vi "Write Graph-Chart Plot Names.vi"(8 "error in":errorcluster, 10 "Value":string[](array[string]), 11 "Graph / Chart Reference in":refnum<vi>) -> (0 "error out":errorcluster, 3 "Graph / Chart Reference out":refnum<vi>)   [LabVIEW 2020, in "G-Unicode.lvlib"]
uses:
  G-Unicode.lvlib
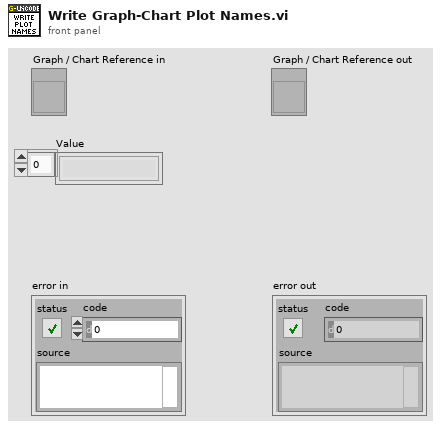
[diagram p1: front panel]
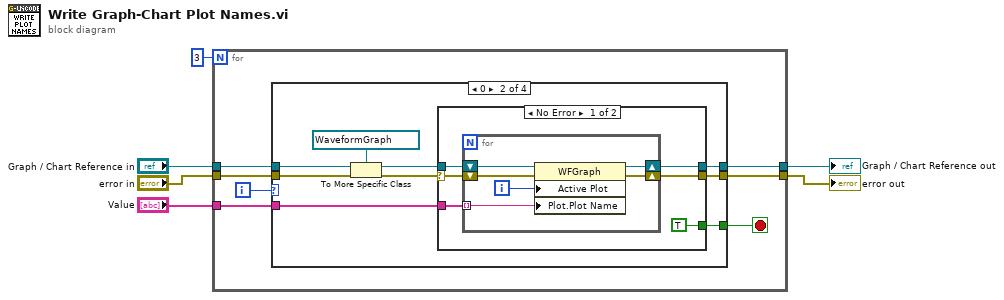
[diagram p0: block diagram]
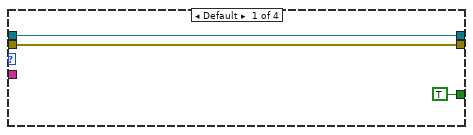
[diagram p2: hidden frame]
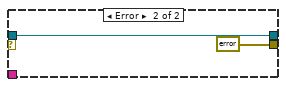
[diagram p3: hidden frame]
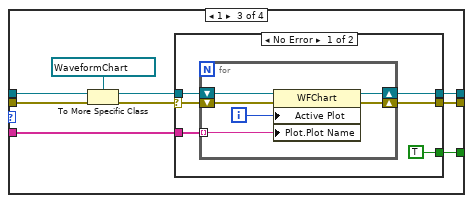
[diagram p4: hidden frame]
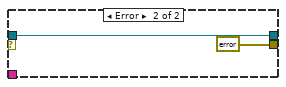
[diagram p5: hidden frame]
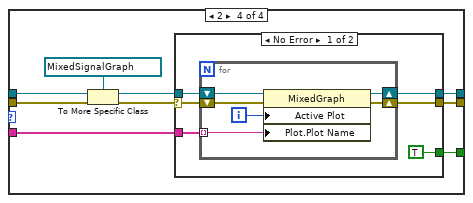
[diagram p6: hidden frame]
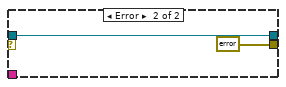
[diagram p7: hidden frame]
diagram:
  n1 = for {
    N: 3 -> [_]
    tunnel: "error in" -> [w13]
    tunnel: [w12] -> w5
    tunnel: [w11] -> w4
    tunnel: "Graph / Chart Reference in" -> [w10]
    tunnel: "Value" -> [w9]
    i -> [w8]
    stop <- w7 stop-if-true
    n2 = case shown="0" w8 {
      tunnel: w13 -> [w15 w20 w43 w66]
      tunnel: [w16 w25 w48 w71] -> w12
      tunnel: [w15 w24 w47 w70] -> w11
      tunnel: w10 -> [w16 w23 w46 w69]
      tunnel: w9 -> [_ w22 w45 w68]
      tunnel: [TRUE w17 w40 w63] -> w7
      frame Default {
      }
      frame 0 {
        n3 = To More Specific Class(target class=refnum<vi> refnum ("Graph / Chart Reference in"), reference=w23, error in=w20) -> (specific class reference=w21:refnum<vi>, error out=w18:errorcluster)
        n4 = case shown="No Error" w18 {
          selector: w18 -> [w27 _]
          tunnel: [w31 w38] -> w25
          tunnel: [w30 errorcluster {"status"=FALSE, "code"=0, "source"=""} ("error IO")] -> w24
          tunnel: w22 -> [w29 _]
          tunnel: w21 -> [w28 w38]
          tunnel: [TRUE _] -> w17
          frame No Error {
            n5 = for {
              tunnel: w29 -> [w33] mode=indexing
              shift-right: [w35] -> w30
              shift-left: w27 -> [w37]
              shift-right: [w36] -> w31
              shift-left: w28 -> [w34]
              i -> [w32]
              n6 = property class="WFGraph"(reference=w34, error in=w37, "Active Plot"=w32, "Plot.Plot Name"=w33) -> (reference out=w36:refnum<vi>, error out=w35:errorcluster)
            }
          }
          frame Error {
          }
        }
      }
      frame 1 {
        n7 = To More Specific Class(target class=refnum<vi> refnum ("Graph / Chart Reference in"), reference=w46, error in=w43) -> (specific class reference=w44:refnum<vi>, error out=w41:errorcluster)
        n8 = case shown="No Error" w41 {
          selector: w41 -> [w50 _]
          tunnel: [w54 w61] -> w48
          tunnel: [w53 errorcluster {"status"=FALSE, "code"=0, "source"=""} ("error IO")] -> w47
          tunnel: w45 -> [w52 _]
          tunnel: w44 -> [w51 w61]
          tunnel: [TRUE _] -> w40
          frame No Error {
            n9 = for {
              tunnel: w52 -> [w56] mode=indexing
              shift-right: [w58] -> w53
              shift-left: w50 -> [w60]
              shift-right: [w59] -> w54
              shift-left: w51 -> [w57]
              i -> [w55]
              n10 = property class="WFChart"(reference=w57, error in=w60, "Active Plot"=w55, "Plot.Plot Name"=w56) -> (reference out=w59:refnum<vi>, error out=w58:errorcluster)
            }
          }
          frame Error {
          }
        }
      }
      frame 2 {
        n11 = To More Specific Class(target class=refnum<vi> refnum ("Graph / Chart Reference in"), reference=w69, error in=w66) -> (specific class reference=w67:refnum<vi>, error out=w64:errorcluster)
        n12 = case shown="No Error" w64 {
          selector: w64 -> [w73 _]
          tunnel: [w77 w84] -> w71
          tunnel: [w76 errorcluster {"status"=FALSE, "code"=0, "source"=""} ("error IO")] -> w70
          tunnel: w68 -> [w75 _]
          tunnel: w67 -> [w74 w84]
          tunnel: [TRUE _] -> w63
          frame No Error {
            n13 = for {
              tunnel: w75 -> [w79] mode=indexing
              shift-right: [w81] -> w76
              shift-left: w73 -> [w83]
              shift-right: [w82] -> w77
              shift-left: w74 -> [w80]
              i -> [w78]
              n14 = property class="MixedGraph"(reference=w80, error in=w83, "Active Plot"=w78, "Plot.Plot Name"=w79) -> (reference out=w82:refnum<vi>, error out=w81:errorcluster)
            }
          }
          frame Error {
          }
        }
      }
    }
  }
  "error out" <- w4
  "Graph / Chart Reference out" <- w5
